vi "Save Image.vi"(8 "error in (no error)":errorcluster, 9 "Path":path, 10 "Image":T1, 11 "Sim Camera Driver in":refnum<class "Sim Camera Driver.lvclass">) -> (0 "error out":errorcluster, 3 "Sim Camera Driver out":refnum<class "Sim Camera Driver.lvclass">)   [LabVIEW 2022 SP3, in "Sim Camera Driver.lvclass"]
uses:
  Sim Camera Driver.lvclass
  <vilib>/vision/Image Controls.llb/IMAQ Image.ctl
  Sim Camera Driver.lvclass/Sim Camera Driver.ctl
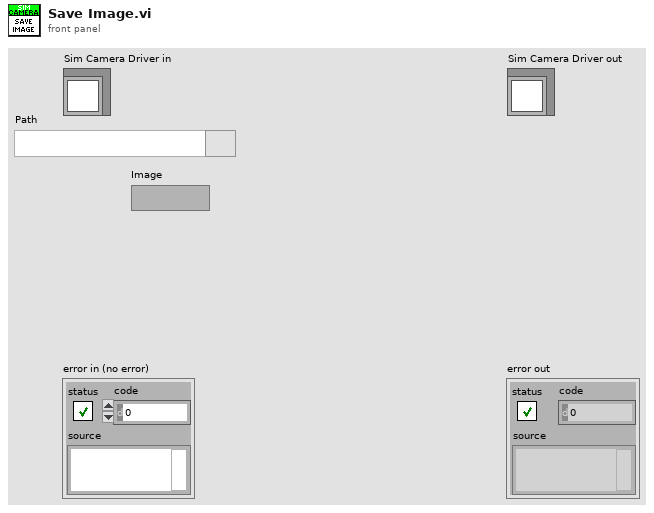
[diagram p1: front panel]
types:
  T1 = typedef "IMAQ Image.ctl" = refnum<image>
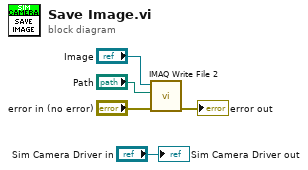
[diagram p0: block diagram]
diagram:
  n1 = call-poly "IMAQ Write File 2"("error in (no error)"="error in (no error)", "File Path"="Path", "Image"="Image") -> ("error out"=→"error out":errorcluster)  [unwired: 7 in, 1 out]
  "Sim Camera Driver out" <- "Sim Camera Driver in"
